vi "Make MDIF file.vi"() -> ()   [LabVIEW 2020]
uses:
  <vilib>/addons/HF Network Analysis/Controls/MDIF Block.ctl
  <vilib>/Utility/Data Type/Type Definitions/Data Type.ctl
  <vilib>/Utility/Data Type/Type Definitions/Memory Info.ctl
  <vilib>/Utility/Data Type/Type Definitions/Memory Type.ctl
  <vilib>/addons/HF Network Analysis/NI_HFNetworkAnalysis.lvlib
  <vilib>/Utility/Data Type/NI_Data Type.lvlib
  <vilib>/addons/HF Network Analysis/Support VIs/Get MDIF Blocks (All).vi
panel:
  out "type string":i16[][](array[numeric])
  out "Array 2":string[](array[string])
  out "Array 7":i32[](array[numeric])
  out "Array Lengths":T1[][](array[typedef])
  out "Array 6":variant[](array[variant])
  out "Array 5":T3[](array[typedef])
  out "Array":string[](array[string])
  out "MDIF Blocks":T4[](array[typedef])
  in  "MDIF File Path":path
  in  "error in (no error)":errorcluster
  in  "file format":string="s2p"
  out "array":string[](array[string])
  in  "Filename has to include:":string="s2p_DUT"
  in  "Save":bool
  in  "SnP File Path":path
  # "Check that the steps are in right order. This script uses filename in alphabetical order."
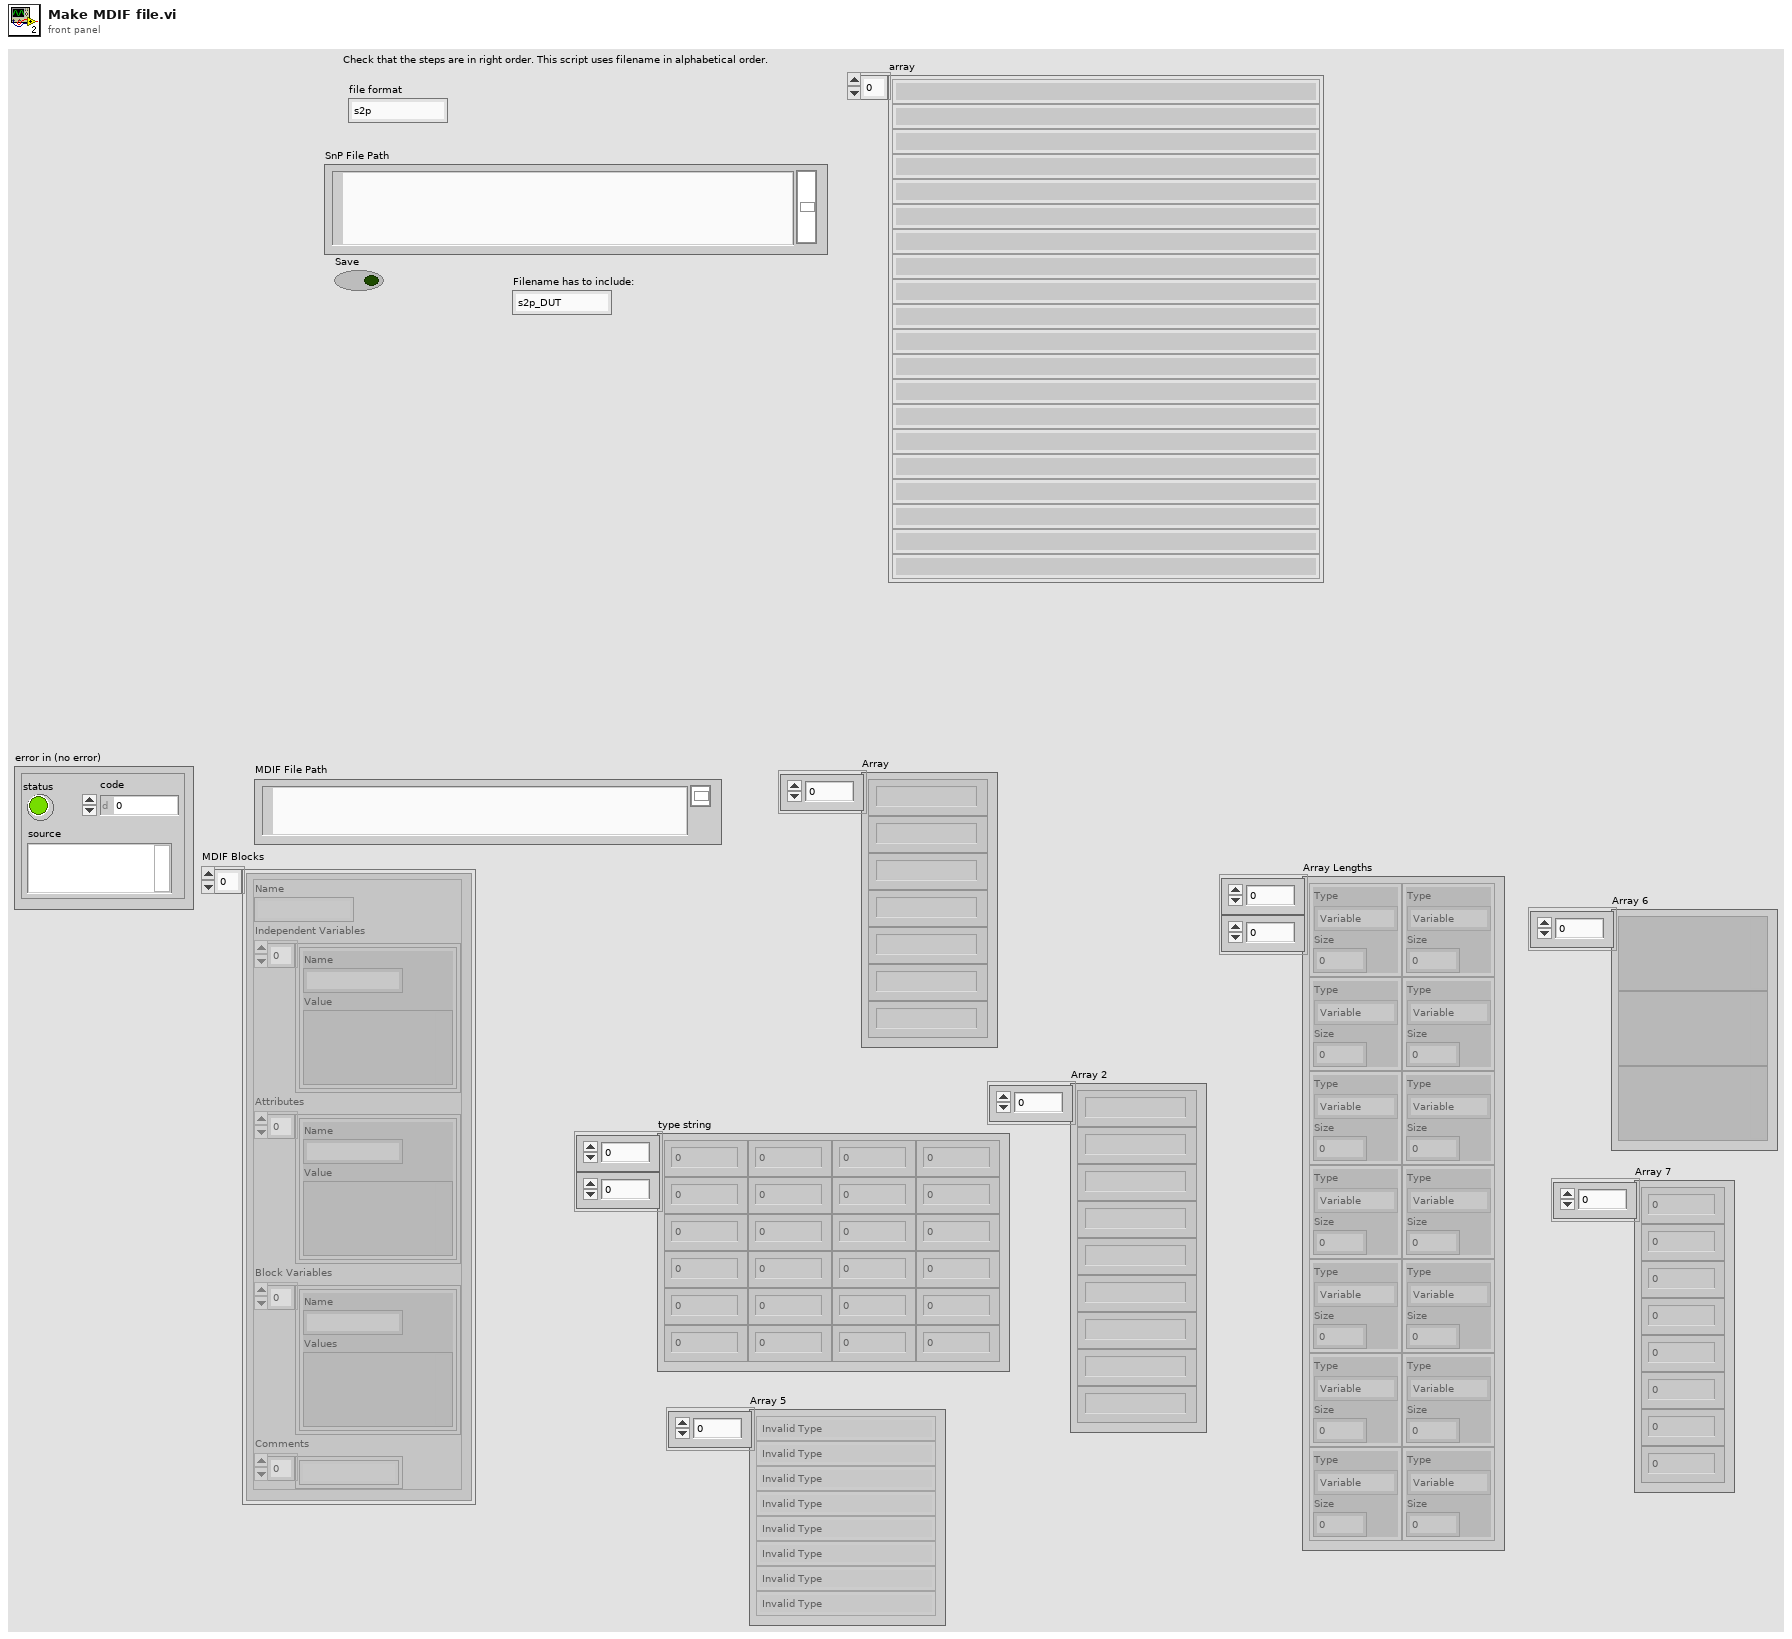
[diagram p1: front panel]
types:
  T1 = typedef "NI_Data Type.lvlib/Memory Info.ctl" = cluster{"Type":T2, "Size":u32}
  T2 = typedef "NI_Data Type.lvlib/Memory Type.ctl" = enum16{"Variable", "Fixed", "Bounded"}
  T3 = typedef "NI_Data Type.lvlib/Data Type.ctl" = enum8{"Invalid Type", "Void", "I8", "I16", "I32", "I64", "U8", "U16", "U32", "U64", "Single Float", "Double Float", "Extended Float", "Single Complex", "Double Complex", "Extended Complex", "Enum U8", "Enum U16", "Enum U32", "Enum U64", "Single Float With Unit", "Double Float With Unit", "Extended Float With Unit", "Single Complex with Unit", "Double Complex with Unit", "Extended Complex with Unit", "Boolean", "String", "Path", "Picture", "Tag", "Array", "Cluster", "Variant", "LV Variant", "Waveform", "Timestamp", "Digital Waveform", "Digital Data", "ExpressData", "Refnum", "External Data", "VI", "Poly VI", "LabVIEW Class Instance", "Fixed Point", "Set Collection", "Map Collection"}
  T4 = typedef "NI_HFNetworkAnalysis.lvlib/MDIF Block.ctl" = cluster{"Name":string, "Independent Variables":cluster{"Name":string, "Value":variant}[], "Attributes":cluster{"Name":string, "Value":variant}[], "Block Variables":cluster{"Name":string, "Values":variant}[], "Comments":string[]}
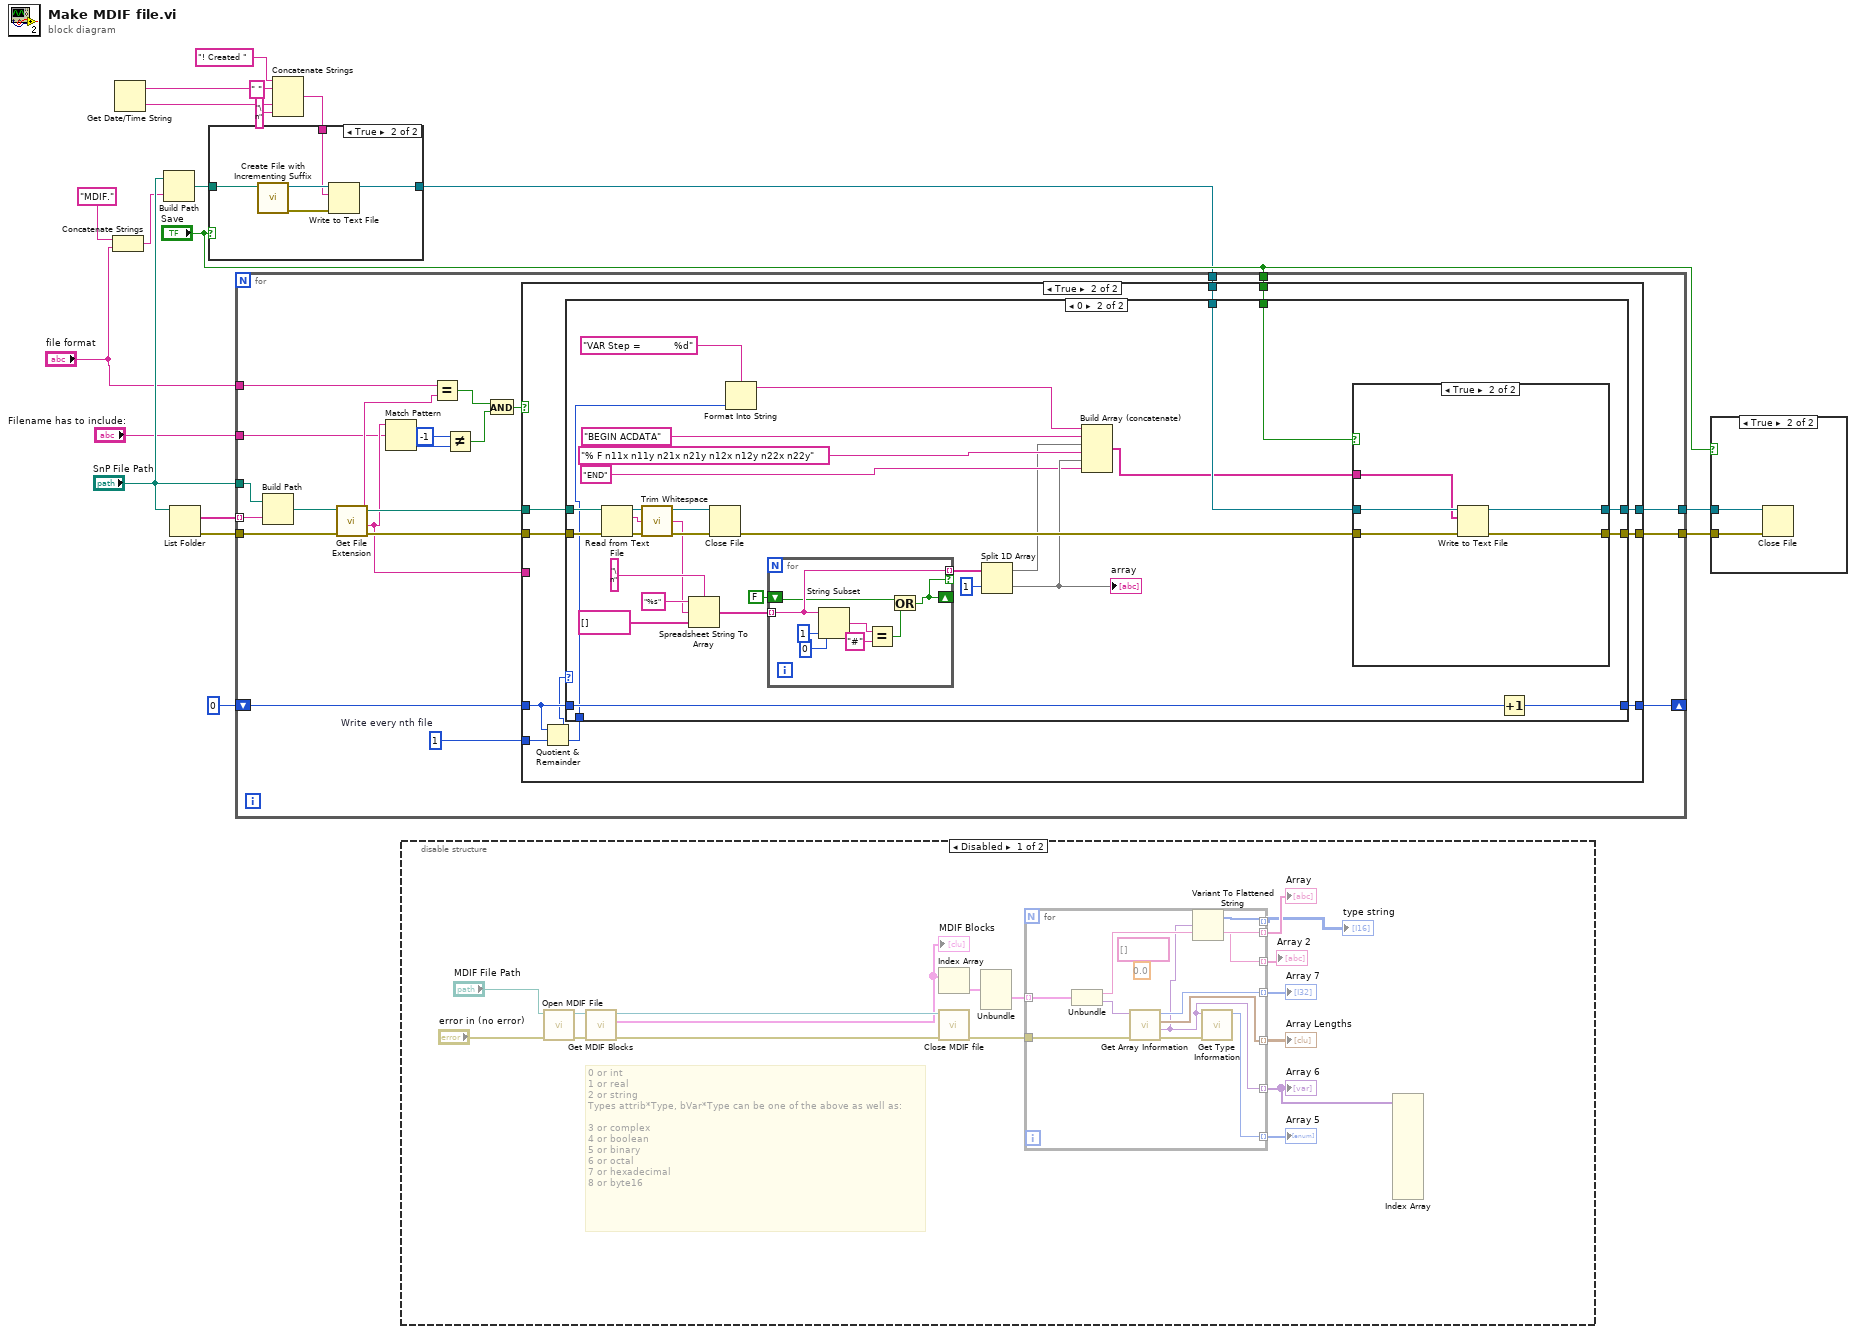
[diagram p0: block diagram]
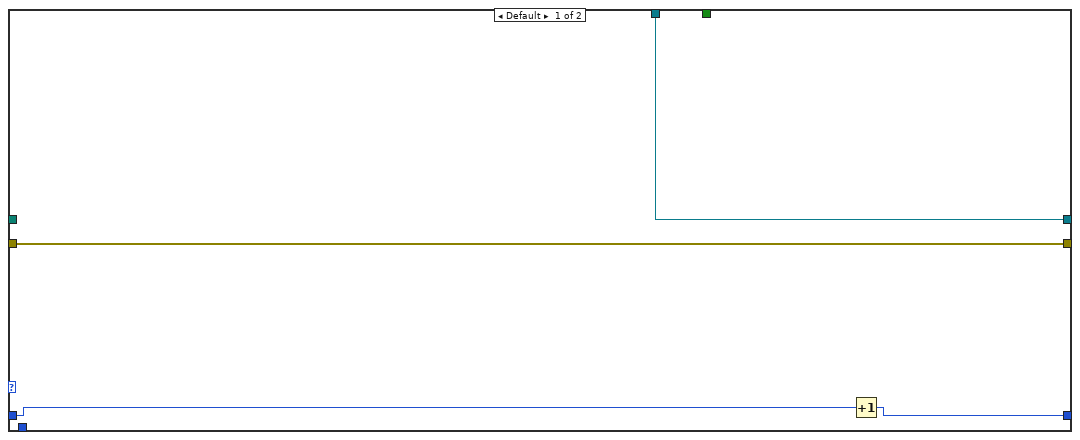
[diagram p6: hidden frame]
diagram:
  n1 = Concatenate Strings("MDIF." ("string"), "file format") -> (w3:string)
  n2 = Get Date/Time String() -> (date string=w7:string, time string=w8:string)  [unwired: 3 in]
  n3 = Build Path(base path="SnP File Path", name or relative path=w3) -> (appended path=w14:path)
  n4 = List Folder(path="SnP File Path") -> (filenames=w19:string[], error out=w17:errorcluster)  [unwired: 3 in, 2 out]
  n5 = Concatenate Strings("! Created ", w7, " " ("string"), w8, "\n" ("string")) -> (w6:string)
  n6 = case shown="True" "Save" {
    tunnel: w14 -> [_ w24]
    tunnel: [_ w21] -> w12
    tunnel: w6 -> [_ w20]
    frame False {
    }
    frame True {
      n7 = call <vilib>:"Create File with Incrementing Suffix.vi"("file path"=w24) -> ("error out"=w23:errorcluster, "refnum out"=w22:refnum<file>)  [unwired: 8 in, 1 out]
      n8 = Write to Text File(file (use dialog)=w22, text=w20, error in=w23) -> (refnum out=w21:refnum<file>)  [unwired: 1 in, 2 out]
    }
  }
  n9 = for {
    tunnel: "SnP File Path" -> [w35]
    tunnel: [w46] -> w10
    tunnel: w17 -> [w40]
    tunnel: w19 -> [w38] mode=indexing
    tunnel: "Filename has to include:" -> [w32]
    shift-right: [w30] -> _
    shift-left: 0 -> [w31]
    tunnel: "Save" -> [w29]
    tunnel: w12 -> [w28]
    tunnel: [w27] -> w11
    tunnel: "file format" -> [w26]
    w25 = 1  # Write every nth file
    n10 = Build Path(base path=w35, name or relative path=w38) -> (appended path=w37:path)
    n11 = call <vilib>:"Get File Extension.vi"("error in (no error)"=w40, "file"=w37) -> ("error out"=w39:errorcluster, "filename without extension"=w33:string, "lowercase file extension"=w43:string, "dup file"=w34:path)  [unwired: 5 in, 1 out]
    n12 = Match Pattern(string=w33, regular expression=w32) -> (offset past match=w36:i32)  [unwired: 1 in, 3 out]
    n13 = Equal?(x=w26, y=w43) -> (x = y?=w44:bool)
    n14 = Not Equal?(x=-1, y=w36) -> (x != y?=w45:bool)
    n15 = And(x=w44, y=w45) -> (x .and. y?=w41:bool)
    n16 = case shown="True" w41 {
      tunnel: w34 -> [_ w60]
      tunnel: [w49 w56] -> w46
      tunnel: w39 -> [w49 w59]
      tunnel: w33 -> [_ _]
      tunnel: w31 -> [w48 w53]
      tunnel: [w48 w58] -> w30
      tunnel: w29 -> [_ w57]
      tunnel: w28 -> [w47 w55]
      tunnel: [w47 w54] -> w27
      tunnel: w25 -> [_ w50]
      frame False {
      }
      frame True {
        n17 = Quotient & Remainder(x=w53, y=w50) -> (x-y*floor(x/y)=w52:i32, floor(x/y)=w51:i32)
        n18 = case shown="0" w52 {
          tunnel: w60 -> [_ w93]
          tunnel: w59 -> [w62 w92]
          tunnel: [w63 w86] -> w58
          tunnel: w57 -> [_ w85]
          tunnel: [w62 w83] -> w56
          tunnel: w55 -> [w61 w82]
          tunnel: [w61 w81] -> w54
          tunnel: w53 -> [w64 w66]
          tunnel: w51 -> [_ w65]
          frame Default {
            n19 = Increment(x=w64) -> (x+1=w63:i32)
          }
          frame 0 {
            n20 = Read from Text File(file (use dialog)=w93, error in=w92) -> (refnum out=w88:refnum<file>, text=w69:string, error out=w89:errorcluster)  [unwired: 2 in, 1 out]
            n21 = call <vilib>:"Trim Whitespace.vi"("string"=w69) -> ("trimmed string"=w68:string)  [unwired: 1 in]
            n22 = Spreadsheet String To Array(delimiter (Tab)="\n", format string="%s", spreadsheet string=w68, array type (2D Dbl)=string[] []) -> (array=w80:string[])
            n23 = Close File(refnum=w88, error in=w89) -> (error out=w84:errorcluster)  [unwired: 1 out]
            n24 = Format Into String(format string="VAR Step =           %d", w65) -> (resulting string=w75:string)  [unwired: 2 in, 1 out]
            n25 = for {
              tunnel: w80 -> [w97] mode=indexing
              tunnel: [w97] -> w77 mode=indexing if=w94
              shift-right: [w94] -> _
              shift-left: FALSE -> [w95]
              n26 = String Subset(string=w97, offset (0)=0, length (rest)=1 ("length (rest)")) -> (substring=w99:string)
              n27 = Equal?(x=w99, y="#") -> (x = y?=w96:bool)
              n28 = Or(x=w95, y=w96) -> (x .or. y?=w94:bool)
            }
            n29 = Split 1D Array(array=w77, index=1) -> (first subarray=w67:string[], second subarray=w72:string[])
            "array" <- w72
            n30 = Build Array (concatenate)(w75, "BEGIN ACDATA", w67, "% F n11x n11y n21x n21y n12x n12y n22x n22y", w72, "END") -> (w70:string[])
            n31 = case shown="True" w85 {
              tunnel: w84 -> [w103 w108]
              tunnel: [w103 w106] -> w83
              tunnel: w82 -> [w102 w107]
              tunnel: [w102 w105] -> w81
              tunnel: w70 -> [_ w104]
              frame False {
              }
              frame True {
                n32 = Write to Text File(file (use dialog)=w107, text=w104, error in=w108) -> (refnum out=w105:refnum<file>, error out=w106:errorcluster)  [unwired: 1 in, 1 out]
              }
            }
            n33 = Increment(x=w66) -> (x+1=w86:i32)
          }
        }
      }
    }
  }
  n34 = disable-structure shown="Disabled" {
    frame Disabled {
      # "0 or int\n1 or real\n2 or string\nTypes attrib*Type, bVar*Type can be one of the above as well as:\n\n3 or complex\n4 or boolean\n5 or binary\n6 or octal\n7 or hexadecimal\n8 or byte16"
      n35 = call <vilib>:"Open MDIF File.vi"("error in (no error)"="error in (no error)", "MDIF File Path"="MDIF File Path") -> ("error out"=w124:errorcluster, "MDIF reference out"=w125:refnum<k24>)  [unwired: 8 in]
      n36 = call-poly <vilib>:"Get MDIF Blocks.vi"("error in (no error)"=w124, "MDIF reference in"=w125) -> ("error out"=w122:errorcluster, "MDIF Blocks"=w119:T4[], "MDIF reference out"=w123:refnum<k24>)  [unwired: 7 in]
      "MDIF Blocks" <- w119
      n37 = Index Array(array=w119) -> (element=w118:T4)  [unwired: 1 in]
      n38 = call <vilib>:"Close MDIF file.vi"("error in (no error)"=w122, "MDIF reference in"=w123) -> ("error out"=w112:errorcluster)  [unwired: 9 in]
      n39 = Unbundle(w118) -> ("Block Variables"=w117:cluster{"Name":string, "Values":variant}[])  [unwired: 4 out]
      n40 = for {
        tunnel: w117 -> [w136] mode=indexing
        tunnel: [w135] -> w116 mode=indexing
        tunnel: [w128] -> w109 mode=indexing
        tunnel: [w134] -> w115 mode=indexing
        tunnel: [w133] -> w113 mode=indexing
        tunnel: [w132] -> w114 mode=indexing
        tunnel: [w126] -> w111 mode=indexing
        tunnel: w112 -> [w130]
        tunnel: [w127] -> w110 mode=indexing
        (unwired) 0.0
        (unwired) string[] []
        n41 = Unbundle(w136) -> ("Name"=w135:string, "Values"=w129:variant)
        n42 = call <vilib>:"Get Array Information.vi"("error in (no error)"=w130, "variant"=w129) -> ("error out"=w131:errorcluster, "array element data type"=w126:variant, "array lengths"=w132:T1[], "number of dimensions"=w133:i32)  [unwired: 6 in]
        n43 = Variant To Flattened String(Variant=w126) -> (data string=w128:string, 1:w127:i16[])
        n44 = call <vilib>:"Get Type Information.vi"("error in (no error)"=w131, "variant"=w126) -> ("type"=w134:T3)  [unwired: 5 in, 4 out]
      }
      "Array" <- w116
      "Array 5" <- w115
      "Array 6" <- w111
      "Array Lengths" <- w114
      "Array 7" <- w113
      "Array 2" <- w109
      "type string" <- w110
      n45 = Index Array(array=w111) -> ()  [unwired: 11 in, 11 out]
    }
    frame Enabled {
    }
  }
  n46 = case shown="True" "Save" {
    tunnel: w11 -> [_ w138]
    tunnel: w10 -> [_ w137]
    frame False {
    }
    frame True {
      n47 = Close File(refnum=w138, error in=w137) -> ()  [unwired: 2 out]
    }
  }
